vi "总氮微站质控流程.vi"(6 "队列输入TN":refnum<queue>, 9 "总氮":bool, 10 "总氮量程切换":enum32{"H", "L", "AUTO"}(ring)=enum."AUTO") -> (3 "布尔":bool)   [LabVIEW 2016, in "质控单元.lvlib"]
panel:
  out "总氮中断报警":bool
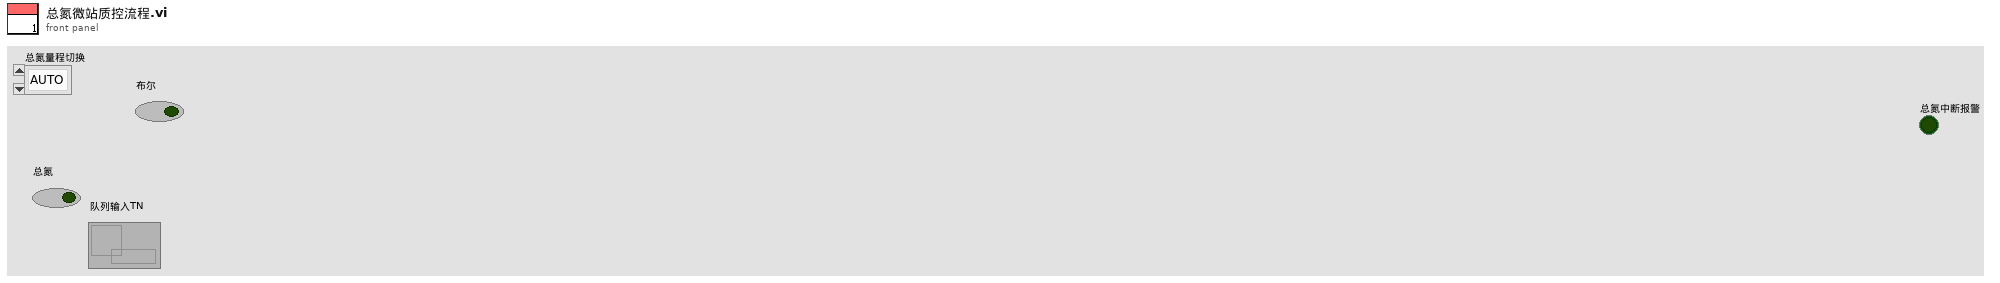
[diagram p1: front panel]
types:
  T1 = enum16{"待机", "启动氨氮水样", "氨氮测量中", "启动氨氮加标", "启动氨氮加标回收", "氨氮加标回收测量中", "启动总氮水样", "总氮测量中", "启动总氮加标", "启动总氮加标回收", "总氮加标回收测量中", "启动总磷水样", "总磷水样测量中", "启动总磷加标", "启动总磷加标回收", "总磷加标回收测量中", "结束"}
  T2 = cluster{"站号":u16, "量程切换":enum32{"H", "L", "AUTO"}, "控制命令":enum16{"启动测量", "标样核查", "零点核查", "跨度核查", "空白测试", "平行样测试", "加标回收", "空白校准", "标样校准", "初始化（清洗）", "停止测试", "仪器重启", "校时", "模式设置", "测量间隔设置"}, "模式设置":enum16{"待机", "连续模式", "周期模式", "定点模式", "受控模式", "手动模式"}, "测量间隔":u16}
  T3 = cluster{"时间标识":timestamp, "设备":string, "日志信息":string}
  T4 = cluster{"系统时间":timestamp, "工作状态":enum16{"空闲", "水样测试", "标样核查", "零点核查", "跨度核查", "空白测试", "平行样测试", "加标回收", "空白校准", "标样校准", "初始化（清洗）"}, "测量模式":enum16{"待机", "连续模式", "周期模式", "定点模式", "受控模式", "手动模式"}, "告警代码":enum16{"无告警", "缺试剂告警", "缺水样告警", "缺蒸馏水告警", "缺标液告警", "仪表漏液告警", "标定异常告警", "超量程告警", "加热异常", "低试剂预警", "超上限告警", "超下限告警", "仪表内部其他异常", "滴定异常告警", "电极异常告警", "量程切换告警", "参数设置告警", "PH电极电位异常", "电导率电极异常", "浊度光度异常", "溶解氧电极异常", "溶解氧光强异常", "温度异常告警", "PH异常告警", "溶解氧异常告警", "电导率异常告警", "浊度异常告警", "叶绿素异常告警", "藻密度异常告警", "蓝绿藻异常告警", "ORP异常告警", "氨氮异常告警", "清洁刷异常告警", "SD卡异常告警", "蓝牙异常告警", "Wifi异常告警", "流程异常告警"}, "故障代码":enum16{"无故障", "电机故障", "温度故障", "通讯故障", "滴定故障"}, "日志代码":u16, "软件版本":u16, "F0":sgl, "F1":sgl, "F2":sgl, "F3":sgl, "T":sgl, "H":sgl, "id":u16, "flowid":u16, "量程":u16, "总磷控温温度1":sgl, "营养盐控温温度2":sgl, "ADC":sgl}
  T5 = enum16{"空闲", "水样测试", "标样核查", "零点核查", "跨度核查", "空白测试", "平行样测试", "加标回收", "空白校准", "标样校准", "初始化（清洗）"}
  T6 = cluster{"因子编码":u32, "单位":u16, "标样参考值":sgl, "水样数据时间":timestamp, "水样实测值":sgl, "水样数据标识":string, "标样数据时间":timestamp, "标样实测值":sgl, "标样数据标识":string, "空白数据时间":timestamp, "空白实测值":sgl, "空白数据标识":string, "零点核查数据时间":timestamp, "零点核查实测值":sgl, "零点核查数据标识":string, "跨度核查数据时间":timestamp, "跨度核查实测值":sgl, "跨度核查数据标识":string, "加标回收数据时间":timestamp, "加标回收实测值":sgl, "加标回收数据标识":string, "平行样数据时间":timestamp, "平行样实测值":sgl, "平行样数据标识":string}
  T7 = cluster{"量程":dbl, "检出限":dbl, "加标前水样浓度":dbl, "加标后水样浓度":dbl, "加标水杯定容体积":dbl, "加标母液浓度":dbl, "加标体积":dbl, "加标回收率":dbl}
  T8 = cluster{"氨氮":u8, "总磷":u8, "总氮":u8, "CODMn":u8, "CODCr":u8}
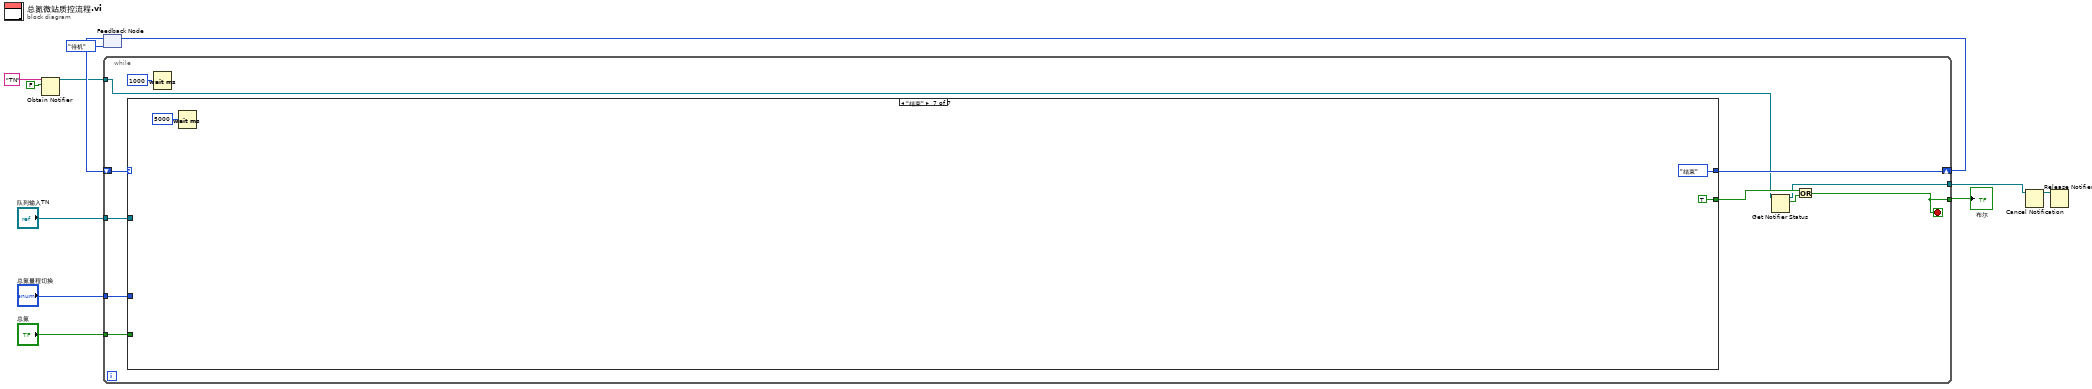
[diagram p0: block diagram]
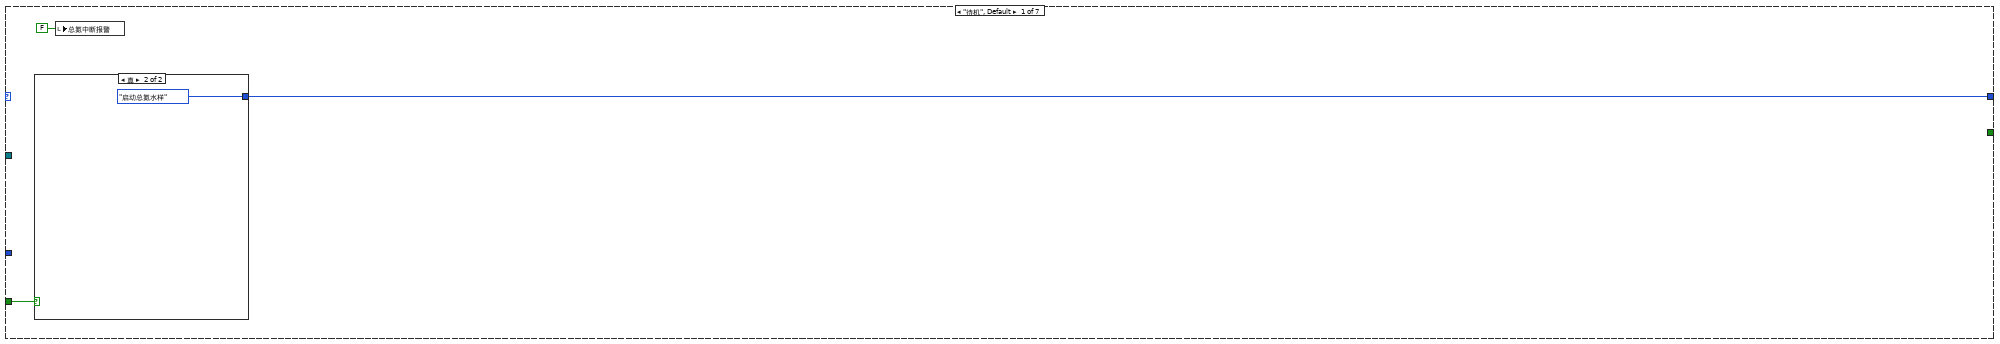
[diagram p2: hidden frame]
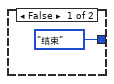
[diagram p3: hidden frame]
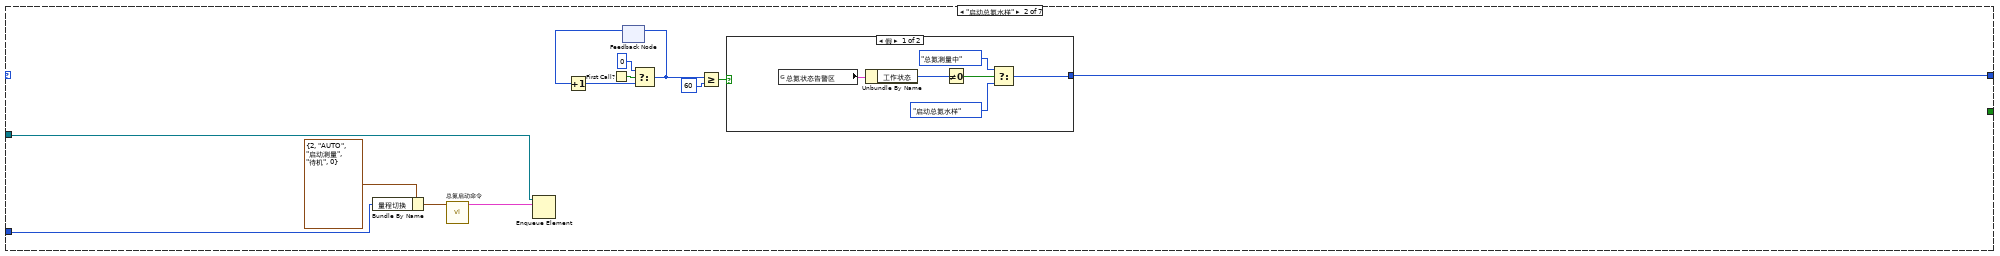
[diagram p4: hidden frame]
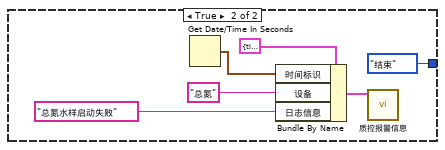
[diagram p5: hidden frame]
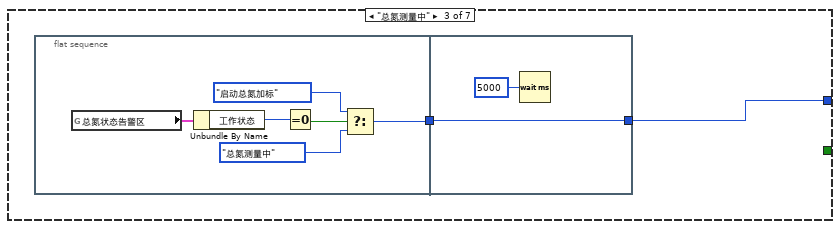
[diagram p6: hidden frame]
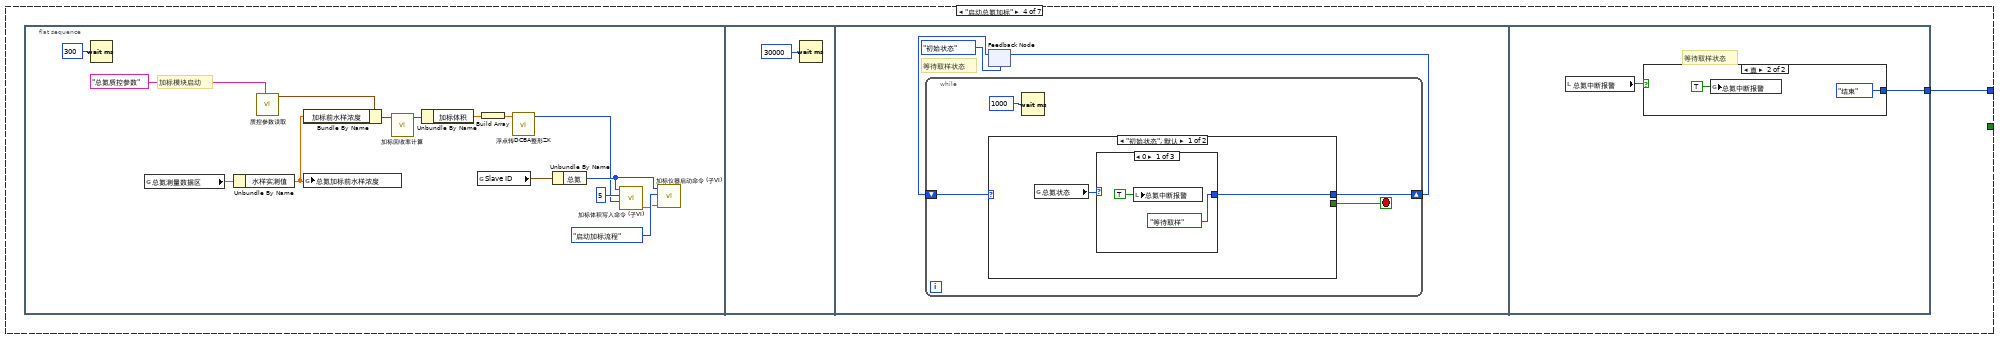
[diagram p7: hidden frame]
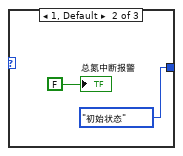
[diagram p8: hidden frame]
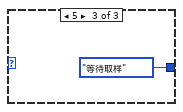
[diagram p9: hidden frame]
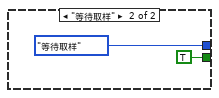
[diagram p10: hidden frame]
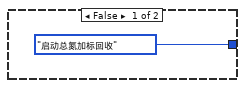
[diagram p11: hidden frame]
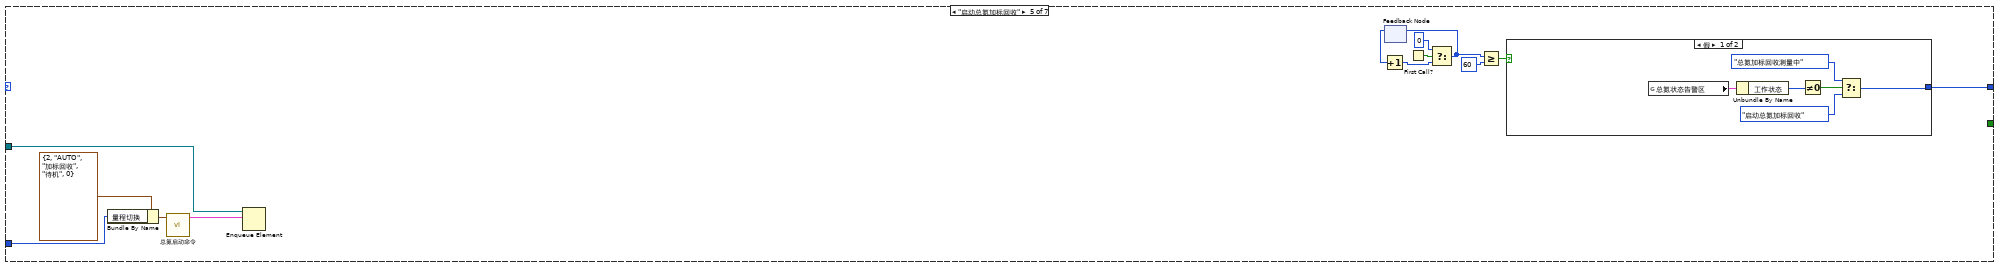
[diagram p12: hidden frame]
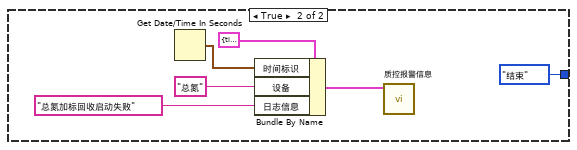
[diagram p13: hidden frame]
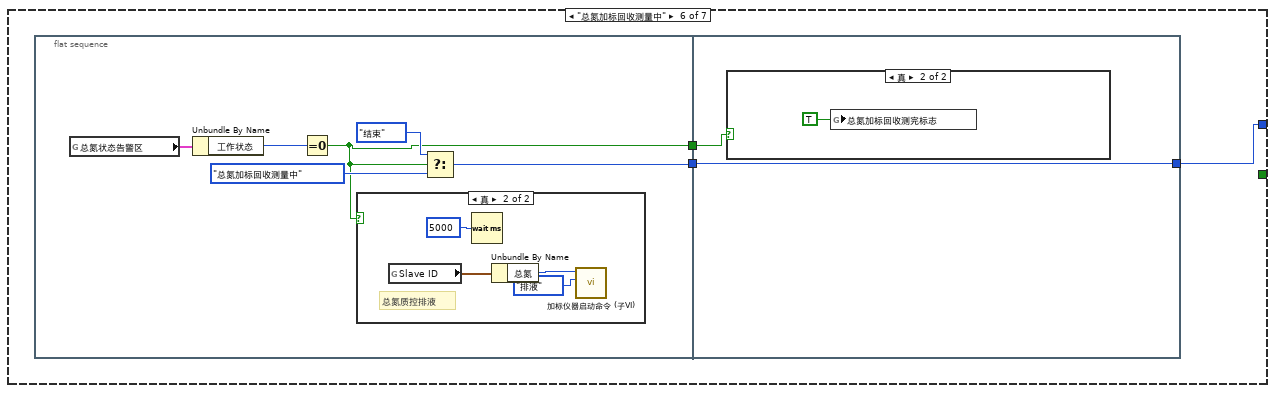
[diagram p14: hidden frame]
diagram:
  n1 = Obtain Notifier(name (unnamed)="TN" ("名称（未命名）"), notification data type=FALSE) -> (notifier out=w3:refnum<notifier>)  [unwired: 2 in, 2 out]
  n2 = feedback #1(T1."待机") -> (w6:T1)
  n3 = while {
    tunnel: "队列输入TN" -> [w21]
    tunnel: "总氮量程切换" -> [w20]
    tunnel: "总氮" -> [w23]
    tunnel: [w15] -> w11
    shift-right: [w22] -> w9
    shift-left: w6 -> [w19]
    tunnel: w3 -> [w13]
    tunnel: [w14] -> w1
    stop <- w15 stop-if-true
    n4 = case shown="\"结束\"" w19 {
      tunnel: [w26 w41 w54 w64 w107 w128 T1."结束"] -> w22
      tunnel: [_ _ _ _ _ _ TRUE] -> w16
      tunnel: w23 -> [w25 _ _ _ _ _ _]
      tunnel: w21 -> [_ w40 _ _ w106 _ _]
      tunnel: w20 -> [_ w39 _ _ w103 _ _]
      frame "待机", Default {
        n5 = case shown="真" w25 {
          tunnel: [T1."结束" T1."启动总氮水样"] -> w26
          frame False {
          }
          frame True {
          }
        }
        n6 = local write "总氮中断报警"(FALSE ("氨氮中断报警")) -> ()
      }
      frame "启动总氮水样" {
        n7 = Bundle By Name(cluster=T2 {"站号"=2, "量程切换"=enum."AUTO", "控制命令"=enum."启动测量", "模式设置"=enum."待机", "测量间隔"=0} ("参数"), "量程切换"=w39) -> (w31:T2)
        n8 = call "总氮启动命令.vi"("参数"=w31) -> ("启动命令"=w29:cluster{"命令":string, "data":variant})  [unwired: 10 in]
        n9 = Enqueue Element(queue=w40, element=w29) -> ()  [unwired: 2 in, 3 out]
        n10 = First Call?() -> (First Call?: T/F=w37:bool)
        n11 = feedback #2() -> (w36:i32)  [unwired: 1 in]
        n12 = Increment(x=w36) -> (x+1=w35:i32)
        n13 = Select(t=0, s=w37, f=w35) -> (s? t:f=w34:i32)
        n14 = feedback-in #2(w34) -> ()
        n15 = Greater Or Equal?(x=w34, y=60) -> (x >= y?=w32:bool)
        n16 = case shown="假" w32 {
          tunnel: [w46 T1."结束"] -> w41
          frame False {
            n17 = global read "与总氮交互全局.vi" "总氮状态告警区"() -> (w43:T4)
            n18 = Unbundle By Name(w43) -> ("工作状态"=w42:T5)
            n19 = Not Equal To 0?(x=w42) -> (x != 0?=w47:bool)
            n20 = Select(t=T1."总氮测量中", s=w47, f=T1."启动总氮水样") -> (s? t:f=w46:T1)
          }
          frame True {
            n21 = Get Date/Time In Seconds() -> (seconds since 1Jan1904=w53:timestamp)
            n22 = Bundle By Name(cluster=T3 {"时间标识"=timestamp(0 s since 1904-01-01), "设备"="", "日志信息"=""} ("data in"), "时间标识"=w53, "设备"="总氮", "日志信息"="总氮水样启动失败") -> (w48:T3)
            n23 = call "质控报警信息.vi"("data in"=w48) -> ()  [unwired: 10 in, 1 out]
          }
        }
      }
      frame "总氮测量中" {
        n24 = flat-sequence {
          tunnel: [w56] -> w55
          tunnel: w55 -> [w62]
          tunnel: [w62] -> w54
          frame #0 {
            n25 = global read "与总氮交互全局.vi" "总氮状态告警区"() -> (w61:T4)
            n26 = Unbundle By Name(w61) -> ("工作状态"=w60:T5)
            n27 = Equal To 0?(x=w60) -> (x = 0?=w59:bool)
            n28 = Select(t=T1."启动总氮加标", s=w59, f=T1."总氮测量中") -> (s? t:f=w56:T1)
          }
          frame #1 {
            n29 = Wait (ms)(milliseconds to wait=u32 5000 ("等待时间（毫秒）")) -> ()  [unwired: 1 out]
          }
        }
      }
      frame "启动总氮加标" {
        n30 = flat-sequence {
          tunnel: [w98] -> w64
          frame #0 {
            # "加标模块启动"
            n31 = Wait (ms)(milliseconds to wait=u32 300 ("等待时间（毫秒）")) -> ()  [unwired: 1 out]
            n32 = global read "与总氮交互全局.vi" "总氮测量数据区"() -> (w72:T6)
            n33 = Unbundle By Name(w72) -> ("水样实测值"=w74:sgl)
            n34 = call "质控参数读取.vi"("section"="总氮质控参数") -> ("参数"=w77:T7)  [unwired: 9 in, 1 out]
            n35 = Bundle By Name(cluster=w77, "加标前水样浓度"=w74) -> (w78:T7)
            n36 = global write "水样浓度全局.vi" "总氮加标前水样浓度"(w74) -> ()
            n37 = call "加标回收率计算.vi"("参数"=w78) -> ("参数 out"=w76:T7)  [unwired: 9 in, 1 out]
            n38 = Unbundle By Name(w76) -> ("加标体积"=w75:dbl)
            n39 = global read "断电保存全局.vi" "Slave ID"() -> (w69:T8)
            n40 = Build Array(w75) -> (w71:dbl[])
            n41 = call "浮点转DCBA整形ZK.vi"("浮点数"=w71) -> ("DCBA整形输出"=w65:u16[])  [unwired: 10 in]
            n42 = Unbundle By Name(w69) -> ("总氮"=w70:u8)
            n43 = call "加标体积写入命令 (子VI).vi"("values"=w65, "starting address"=u16 5, "Slave ID"=w70) -> ("错误输出"=w67:errorcluster)  [unwired: 8 in]
            n44 = call "加标仪器启动命令 (子VI).vi"("错误输入（无错误）"=w67, "启动命令"=enum16{"启动水样流程", "启动加标流程", "排液", "停止"}."启动加标流程", "仪器"=w70) -> ()  [unwired: 8 in, 1 out]
          }
          frame #1 {
            n45 = Wait (ms)(milliseconds to wait=u32 30000 ("等待时间（毫秒）")) -> ()  [unwired: 1 out]
          }
          frame #2 {
            # "等待取样状态"
            n46 = feedback #3(enum16{"初始状态", "等待取样"}."初始状态") -> (w82:enum16{"初始状态", "等待取样"})
            n47 = while {
              shift-right: [w86] -> w83
              shift-left: w82 -> [w87]
              stop <- w85 stop-if-true
              n48 = case shown="\"初始状态\", 默认" w87 {
                tunnel: [w89 enum16{"初始状态", "等待取样"}."等待取样"] -> w86
                tunnel: [_ TRUE] -> w85
                frame "初始状态", Default {
                  n49 = global read "加标回收状态全局变量.vi" "总氮状态"() -> (w88:u16)
                  n50 = case shown="0" w88 {
                    tunnel: [enum16{"初始状态", "等待取样"}."等待取样" enum16{"初始状态", "等待取样"}."初始状态" enum16{"初始状态", "等待取样"}."等待取样"] -> w89
                    frame 0 {
                      n51 = local write "总氮中断报警"(TRUE ("氨氮中断报警")) -> ()
                    }
                    frame 1, Default {
                      "总氮中断报警" <- FALSE ("总氮中断报警")
                    }
                    frame 5 {
                    }
                  }
                }
                frame "等待取样" {
                }
              }
              n52 = Wait (ms)(milliseconds to wait=u32 1000 ("等待时间（毫秒）")) -> ()  [unwired: 1 out]
            }
            n53 = feedback-in #3(w83) -> ()
          }
          frame #3 {
            # "等待取样状态"
            n54 = local read "总氮中断报警"() -> (w97:bool)
            n55 = case shown="真" w97 {
              tunnel: [T1."启动总氮加标回收" T1."结束"] -> w98
              frame False {
              }
              frame True {
                n56 = global write "质控中断报警全局.vi" "总氮中断报警"(TRUE ("总氮中断报警")) -> ()
              }
            }
          }
        }
      }
      frame "启动总氮加标回收" {
        n57 = Bundle By Name(cluster=T2 {"站号"=2, "量程切换"=enum."AUTO", "控制命令"=enum."加标回收", "模式设置"=enum."待机", "测量间隔"=0} ("参数"), "量程切换"=w103) -> (w105:T2)
        n58 = call "总氮启动命令.vi"("参数"=w105) -> ("启动命令"=w102:cluster{"命令":string, "data":variant})  [unwired: 10 in]
        n59 = Enqueue Element(queue=w106, element=w102) -> ()  [unwired: 2 in, 3 out]
        n60 = feedback #4() -> (w112:i32)  [unwired: 1 in]
        n61 = Increment(x=w112) -> (x+1=w111:i32)
        n62 = First Call?() -> (First Call?: T/F=w113:bool)
        n63 = Select(t=0, s=w113, f=w111) -> (s? t:f=w110:i32)
        n64 = feedback-in #4(w110) -> ()
        n65 = Greater Or Equal?(x=w110, y=60) -> (x >= y?=w108:bool)
        n66 = case shown="假" w108 {
          tunnel: [w118 T1."结束"] -> w107
          frame False {
            n67 = global read "与总氮交互全局.vi" "总氮状态告警区"() -> (w115:T4)
            n68 = Unbundle By Name(w115) -> ("工作状态"=w120:T5)
            n69 = Not Equal To 0?(x=w120) -> (x != 0?=w119:bool)
            n70 = Select(t=T1."总氮加标回收测量中", s=w119, f=T1."启动总氮加标回收") -> (s? t:f=w118:T1)
          }
          frame True {
            n71 = Get Date/Time In Seconds() -> (seconds since 1Jan1904=w126:timestamp)
            n72 = Bundle By Name(cluster=T3 {"时间标识"=timestamp(0 s since 1904-01-01), "设备"="", "日志信息"=""} ("data in"), "时间标识"=w126, "设备"="总氮", "日志信息"="总氮加标回收启动失败") -> (w121:T3)
            n73 = call "质控报警信息.vi"("data in"=w121) -> ()  [unwired: 10 in, 1 out]
          }
        }
      }
      frame "总氮加标回收测量中" {
        n74 = flat-sequence {
          tunnel: [w134] -> w129
          tunnel: [w130] -> w127
          tunnel: [w141] -> w128
          tunnel: w129 -> [w141]
          tunnel: w127 -> [w140]
          frame #0 {
            n75 = global read "与总氮交互全局.vi" "总氮状态告警区"() -> (w131:T4)
            n76 = Unbundle By Name(w131) -> ("工作状态"=w135:T5)
            n77 = Equal To 0?(x=w135) -> (x = 0?=w130:bool)
            n78 = case shown="真" w130 {
              frame False {
              }
              frame True {
                # "总氮质控排液"
                n79 = global read "断电保存全局.vi" "Slave ID"() -> (w137:T8)
                n80 = Wait (ms)(milliseconds to wait=u32 5000 ("等待时间（毫秒）")) -> ()  [unwired: 1 out]
                n81 = Unbundle By Name(w137) -> ("总氮"=w138:u8)
                n82 = call "加标仪器启动命令 (子VI).vi"("启动命令"=enum16{"启动水样流程", "启动加标流程", "排液", "停止"}."排液", "仪器"=w138) -> ()  [unwired: 9 in, 1 out]
              }
            }
            n83 = Select(t=T1."结束", s=w130, f=T1."总氮加标回收测量中") -> (s? t:f=w134:T1)
          }
          frame #1 {
            n84 = case shown="真" w140 {
              frame False {
              }
              frame True {
                n85 = global write "质控测完标志全局 1.vi" "总氮加标回收测完标志"(TRUE) -> ()
              }
            }
          }
        }
      }
      frame "结束" {
        n86 = Wait (ms)(milliseconds to wait=u32 5000 ("等待时间（毫秒）")) -> ()  [unwired: 1 out]
      }
    }
    n87 = Wait (ms)(milliseconds to wait=u32 1000 ("等待时间（毫秒）")) -> ()  [unwired: 1 out]
    n88 = Get Notifier Status(notifier=w13) -> (notifier out=w14:refnum<notifier>, current notification=w17:bool)  [unwired: 1 in, 3 out]
    n89 = Or(x=w16, y=w17) -> (x .or. y?=w15:bool)
  }
  "布尔" <- w11
  n90 = feedback-in #1(w9) -> ()
  n91 = Cancel Notification(0:w1) -> (8:w2:refnum<notifier>)  [unwired: 1 in, 2 out]
  n92 = Release Notifier(notifier=w2) -> ()  [unwired: 2 in, 3 out]
